vi "Rack-Refresh.vi"(8 "error in (no error)":errorcluster) -> (0 "error out":errorcluster, 3 "Data Cluster":T1)   [LabVIEW 2015]
doc: "Refreshes the rack input drivers and returns the most recent results.\n\nData Cluster: latest input readings"
uses:
  Typedefs/InputData cluster.ctl
  Port drivers/DigitalInput-DataCluster.ctl
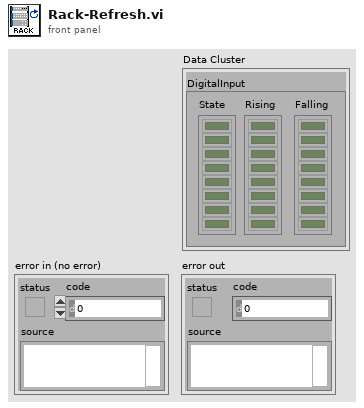
[diagram p1: front panel]
types:
  T1 = typedef "InputData cluster.ctl" = cluster{"DigitalInput":T2}
  T2 = typedef "DigitalInput-DataCluster.ctl" = cluster{"Falling":bool[], "Rising":bool[], "State":bool[]}
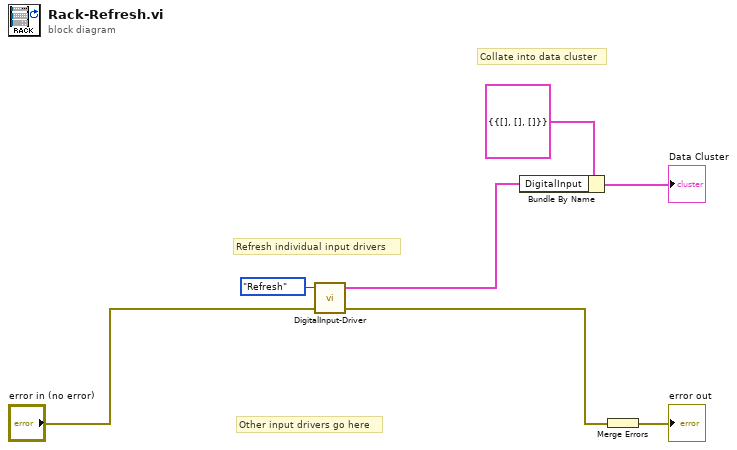
[diagram p0: block diagram]
diagram:
  # "Other input drivers go here"
  # "Collate into data cluster"
  # "Refresh individual input drivers"
  n1 = call "DigitalInput-Driver.vi"("error in (no error)"="error in (no error)", "Command"=enum16{"Refresh", "Start", "Stop"}."Refresh") -> ("error out"=w3:errorcluster, "DigitalInput"=w5:T2)  [unwired: 2 in]
  n2 = Bundle By Name(cluster=T1 {"DigitalInput"={"Falling"=[], "Rising"=[], "State"=[]}} ("Data Cluster"), "DigitalInput"=w5) -> (→"Data Cluster":T1)
  n3 = Merge Errors(w3) -> (→"error out":errorcluster)
